vi "Destroy.vi"(0 "reference in":refnum<class "MyG#G3Templ.lvclass">, 5 "error in (no error)":errorcluster) -> (14 "reference out":refnum<class "MyG#G3Templ.lvclass">, 19 "error out":errorcluster)   [LabVIEW 2020, in "MyG#G3Templ.lvclass"]
doc: "Destructor."
uses:
  MyG#G3Templ.lvclass
  C:/ProjectGSharpDevelopment_2020-3/gsharp/VIPM/Files/vi.lib/addons/_AddQ/G#Object/G#Object.lvclass
  vi.lib/addons/_AddQ/G#Object/G#Object.lvclass
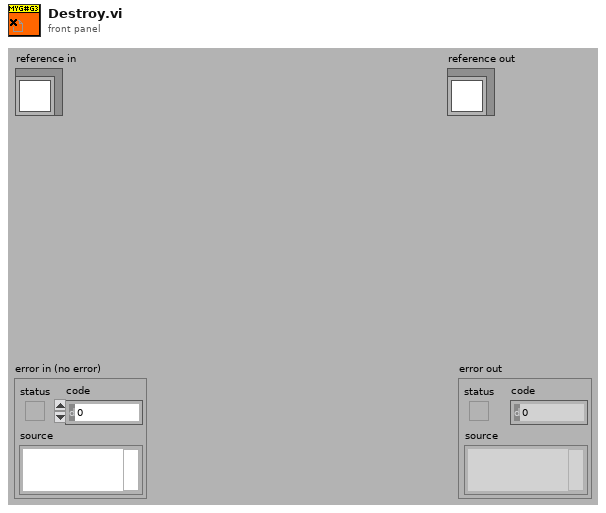
[diagram p1: front panel]
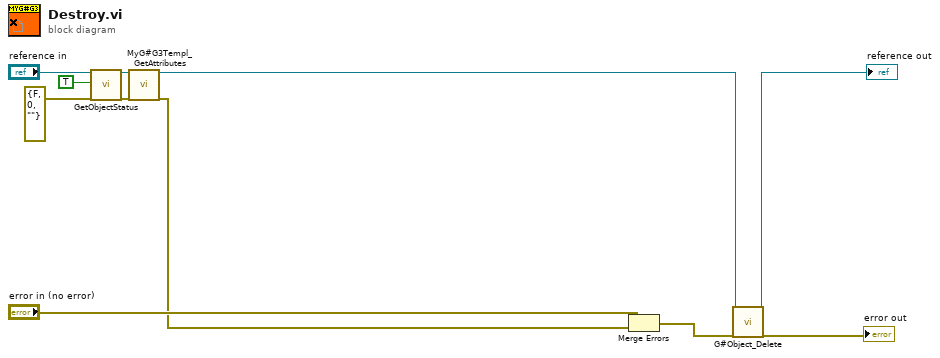
[diagram p0: block diagram]
diagram:
  n1 = call-dynamic "GetObjectStatus.vi"("reference in"="reference in", "simple info (F)"=TRUE ("simple info"), "error in (no error)"=errorcluster {"status"=FALSE, "code"=0, "source"=""}) -> ("reference out"=w6:refnum<class "MyG#G3Templ.lvclass">, "error out"=w4:errorcluster)  [unwired: 5 in, 10 out]
  n2 = call "MyG#G3Templ_GetAttributes.vi"("reference in"=w6, "error in (no error)"=w4) -> ("reference out"=w1:refnum<class "MyG#G3Templ.lvclass">, "error out"=w8:errorcluster)  [unwired: 14 in, 2 out]
  n3 = Merge Errors("error in (no error)", w8) -> (w2:errorcluster)
  n4 = call "G#Object_Delete.vi"("reference in"=w1, "error in (no error)"=w2) -> ("reference out"=→"reference out":refnum<class "MyG#G3Templ.lvclass">, "error out"=→"error out":errorcluster)  [unwired: 16 in]
